vi "CMD Build Bat.vi"(8 "error in (no error)":errorcluster, 11 "batch file":path) -> (0 "error out":errorcluster)   [LabVIEW 2019, in "PostBuildSupport.lvclass"]
uses:
  PostBuildSupport.lvclass
panel:
  out "PID":string
  out "standard output":string
  out "time stamp":timestamp
  in  "stop":bool
  out "Status":string
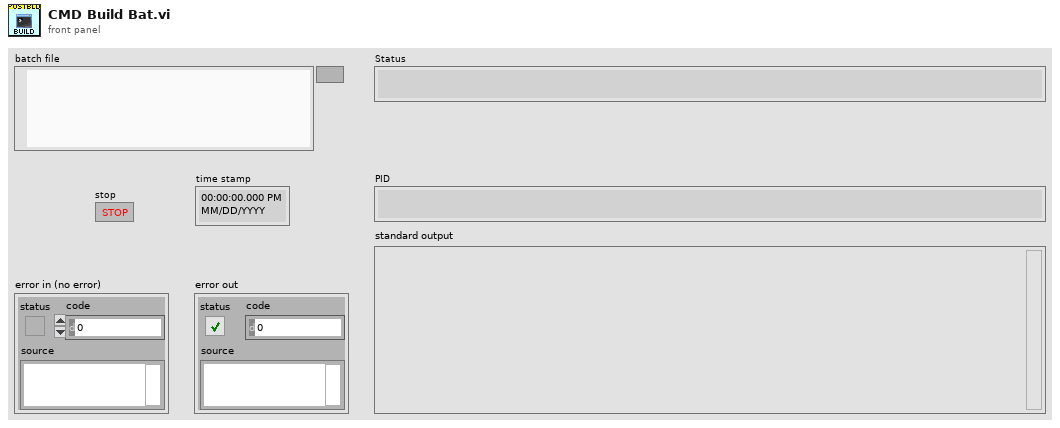
[diagram p1: front panel]
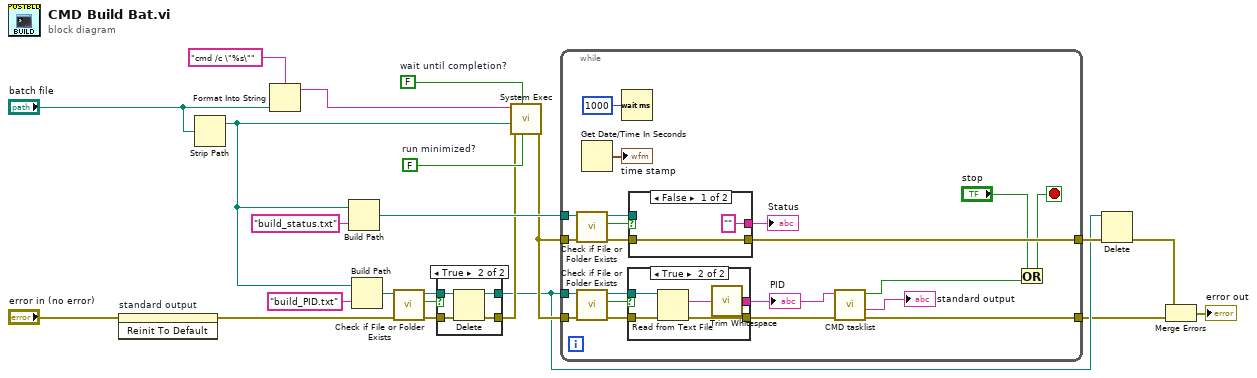
[diagram p0: block diagram]
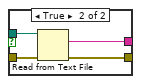
[diagram p2: hidden frame]
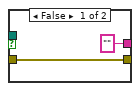
[diagram p3: hidden frame]
diagram:
  w20 = FALSE  # run minimized?
  w21 = FALSE  # wait until completion?
  n1 = invoke on="standard output" class="Str" method="Reinit To Default"(error in="error in (no error)") -> (error out=w7:errorcluster)  [unwired: 2 in, 2 out]
  n2 = Strip Path(path="batch file") -> (stripped path=w2:path)  [unwired: 1 out]
  n3 = Format Into String(format string="cmd /c \"%s\"", "batch file") -> (resulting string=w19:string)  [unwired: 2 in, 1 out]
  n4 = Build Path(base path=w2, name or relative path="build_status.txt") -> (appended path=w17:path)
  n5 = Build Path(base path=w2, name or relative path="build_PID.txt") -> (appended path=w13:path)
  n6 = call <vilib>:"Check if File or Folder Exists.vi"("error in (no error)"=w7, "path"=w13) -> ("error out"=w11:errorcluster, "file or folder exists?"=w10:bool, "dup path"=w12:path)  [unwired: 7 in]
  n7 = case shown="True" w10 {
    tunnel: [w23 w28] -> w14
    tunnel: [w24 w27] -> w8
    tunnel: w12 -> [w24 w26]
    tunnel: w11 -> [w23 w25]
    frame False {
    }
    frame True {
      n8 = Delete(path (use dialog)=w26, error in=w25) -> (deleted path=w27:path, error out=w28:errorcluster)  [unwired: 3 in, 1 out]
    }
  }
  n9 = call <vilib>:"System Exec.vi"("run minimized? (F)"=w20, "wait until completion? (T)"=w21, "error in (no error)"=w14, "working directory"=w2, "command line"=w19) -> ("error out"=w9:errorcluster)  [unwired: 3 in, 3 out]
  n10 = while {
    tunnel: w17 -> [w33]
    tunnel: [w49] -> w15
    tunnel: w8 -> [w40]
    tunnel: w9 -> [w37]
    tunnel: w9 -> [w34]
    tunnel: [w29] -> w4
    stop <- w42 stop-if-true
    n11 = call <vilib>:"Check if File or Folder Exists.vi"("error in (no error)"=w34, "path"=w33) -> ("error out"=w32:errorcluster, "file or folder exists?"=w31:bool, "dup path"=w30:path)  [unwired: 7 in]
    n12 = call <vilib>:"Check if File or Folder Exists.vi"("error in (no error)"=w37, "path"=w40) -> ("error out"=w36:errorcluster, "file or folder exists?"=w39:bool, "dup path"=w41:path)  [unwired: 7 in]
    n13 = Get Date/Time In Seconds() -> (seconds since 1Jan1904=→"time stamp":timestamp)
    n14 = Wait (ms)(milliseconds to wait=u32 1000) -> ()  [unwired: 1 out]
    n15 = case shown="True" w39 {
      tunnel: ["" ("trimmed string") w61] -> w45
      tunnel: w41 -> [_ w60]
      tunnel: w36 -> [w56 w59]
      tunnel: [w56 w58] -> w35
      frame False {
      }
      frame True {
        n16 = Read from Text File(file (use dialog)=w60, error in=w59) -> (text=w62:string, error out=w58:errorcluster)  [unwired: 2 in, 2 out]
        n17 = call <vilib>:"Trim Whitespace.vi"("string"=w62) -> ("trimmed string"=w61:string)  [unwired: 1 in]
      }
    }
    "PID" <- w45
    n18 = case shown="False" w31 {
      tunnel: [w50 w55] -> w49
      tunnel: ["" w54] -> w46
      tunnel: w32 -> [w50 w53]
      tunnel: w30 -> [_ w52]
      frame False {
      }
      frame True {
        n19 = Read from Text File(file (use dialog)=w52, error in=w53) -> (text=w54:string, error out=w55:errorcluster)  [unwired: 2 in, 2 out]
      }
    }
    "Status" <- w46
    n20 = call "CMD tasklist.vi"("error in"=w35, "PID"=w45) -> ("error out"=w29:errorcluster, "output"=→"standard output":string, "Finished"=w44:bool)  [unwired: 6 in, 1 out]
    n21 = Or(x="stop", y=w44) -> (x .or. y?=w42:bool)
  }
  n22 = Delete(path (use dialog)=w8, error in=w15) -> (error out=w5:errorcluster)  [unwired: 3 in, 2 out]
  n23 = Merge Errors(w5, w4) -> (→"error out":errorcluster)
